vi "Fan ADC to RPM calculator (SubVI).vi"(11 "Fan Speed ADC":dbl) -> (3 "Fan Speed RPM":dbl)   [LabVIEW 2024]
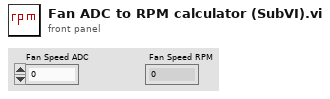
[diagram p1: front panel]
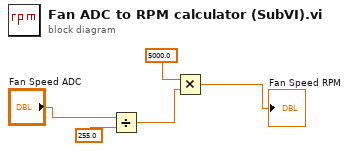
[diagram p0: block diagram]
diagram:
  n1 = Divide(x="Fan Speed ADC", y=255.0) -> (x/y=w3:dbl)
  n2 = Multiply(x=5000.0, y=w3) -> (x*y=→"Fan Speed RPM":dbl)
